vi "configuration methods.vi"() -> (0 "error out":errorcluster, 2 "success?":bool)   [LabVIEW 2013, in "shared memory tests.lvlib"]
uses:
  shared memory tests.lvlib
  module/configuration/shared memory configuration.lvclass
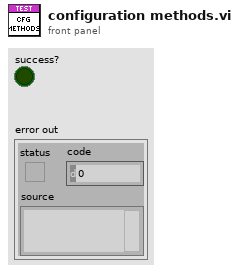
[diagram p1: front panel]
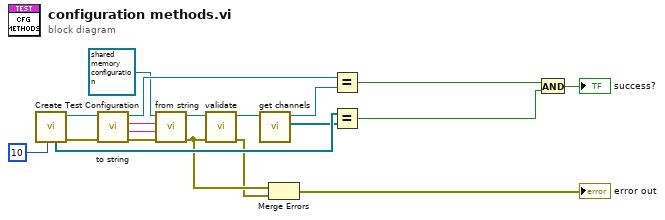
[diagram p0: block diagram]
diagram:
  n1 = call "Create Test Configuration.vi"("number of channels per data type (1)"=10) -> ("error out"=w13:errorcluster, "Module Configuration"=w14:refnum<class "shared memory configuration.lvclass">, "Channels"=w9:refnum<class "TBM channel.lvclass">[])  [unwired: 5 in, 3 out]
  n2 = call-dynamic "to string.vi"("error in"=w13, "shared memory configuration in"=w14) -> ("error out"=w19:errorcluster, "data"=w18:string, "version"=w17:string, "shared memory configuration out"=w11:refnum<class "shared memory configuration.lvclass">)  [unwired: 6 in]
  n3 = call-dynamic "from string.vi"("error in"=w19, "data"=w18, "version"=w17, "shared memory configuration in"=refnum<class "shared memory configuration.lvclass"> refnum ("tag bus configurable plugin module configuration")) -> ("error out"=w7:errorcluster, "shared memory configuration out"=w16:refnum<class "shared memory configuration.lvclass">)  [unwired: 6 in]
  n4 = call-dynamic "validate.vi"("error in"=w7, "shared memory configuration in"=w16) -> ("error out"=w6:errorcluster, "shared memory configuration out"=w15:refnum<class "shared memory configuration.lvclass">)  [unwired: 8 in]
  n5 = call-dynamic "get channels.vi"("shared memory configuration in"=w15) -> ("channels"=w8:refnum<class "TBM channel.lvclass">[], "shared memory configuration out"=w12:refnum<class "shared memory configuration.lvclass">)  [unwired: 9 in]
  n6 = Merge Errors(w7, w6) -> (→"error out":errorcluster)
  n7 = Equal?(x=w11, y=w12) -> (x = y?=w2:bool)
  n8 = Equal?(x=w9, y=w8) -> (x = y?=w3:bool)
  n9 = And(x=w2, y=w3) -> (x .and. y?=→"success?":bool)
